vi "CIC_reconfigure_test.vi"() -> ()   [LabVIEW 2013]
uses:
  <vilib>/Analysis/NI_AALBase.lvlib
panel:
  out "Max 2":fxp<+/-,25,19>
  in  "rate":fxp<+,8,8>
  in  "new rate":bool
  out "Array":bool[](array[boolean])
  out "Max Generated":dbl
  out "Simulated":dbl[](graph)
  in  "stop":bool
  out "Filtered":dbl(graph)
  out "Max":fxp<+/-,25,19>
  out "# of Iterations":i32
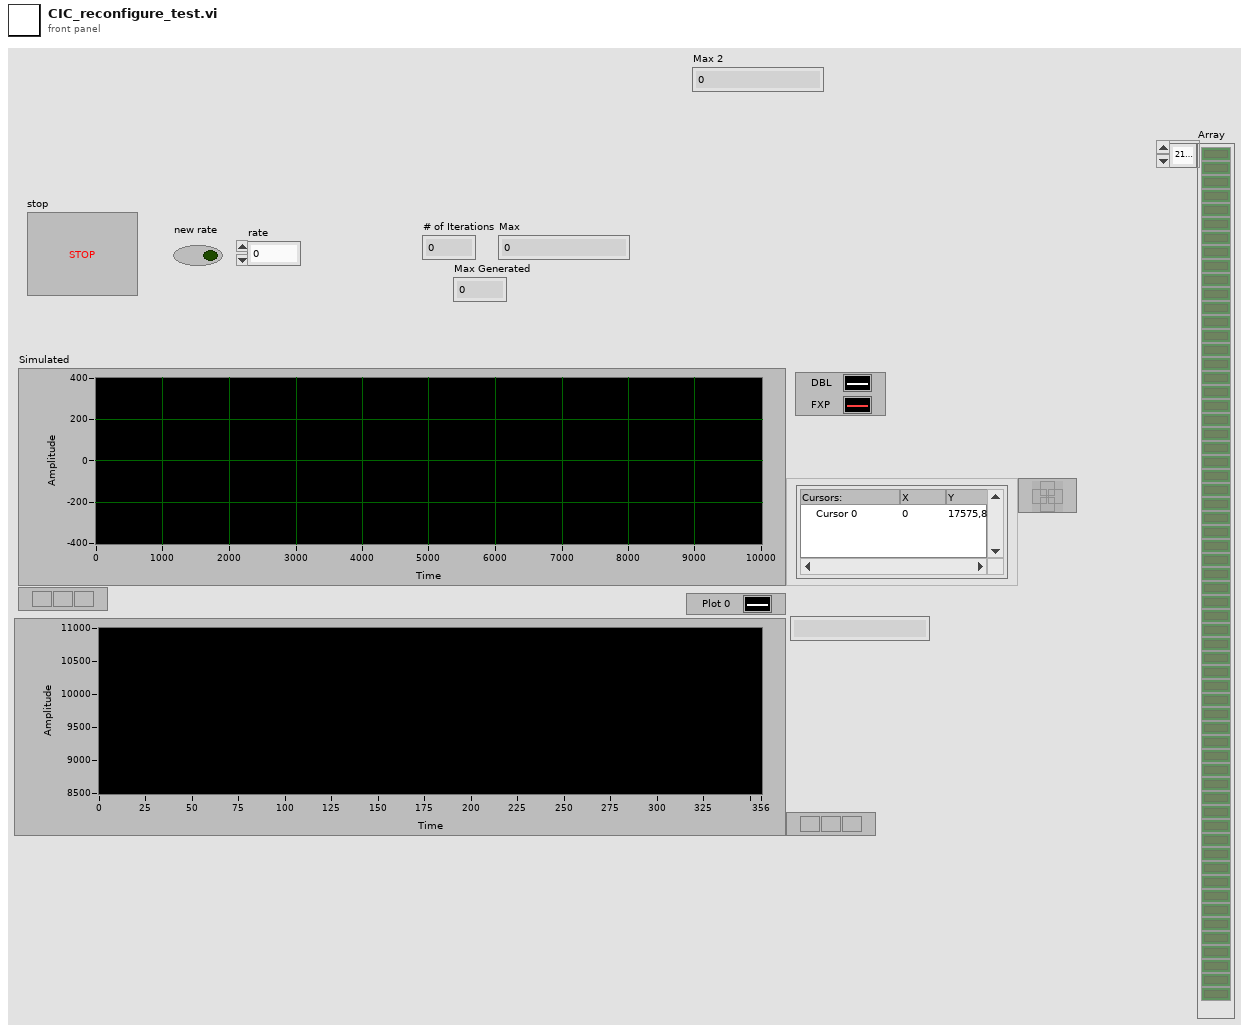
[diagram p1: front panel]
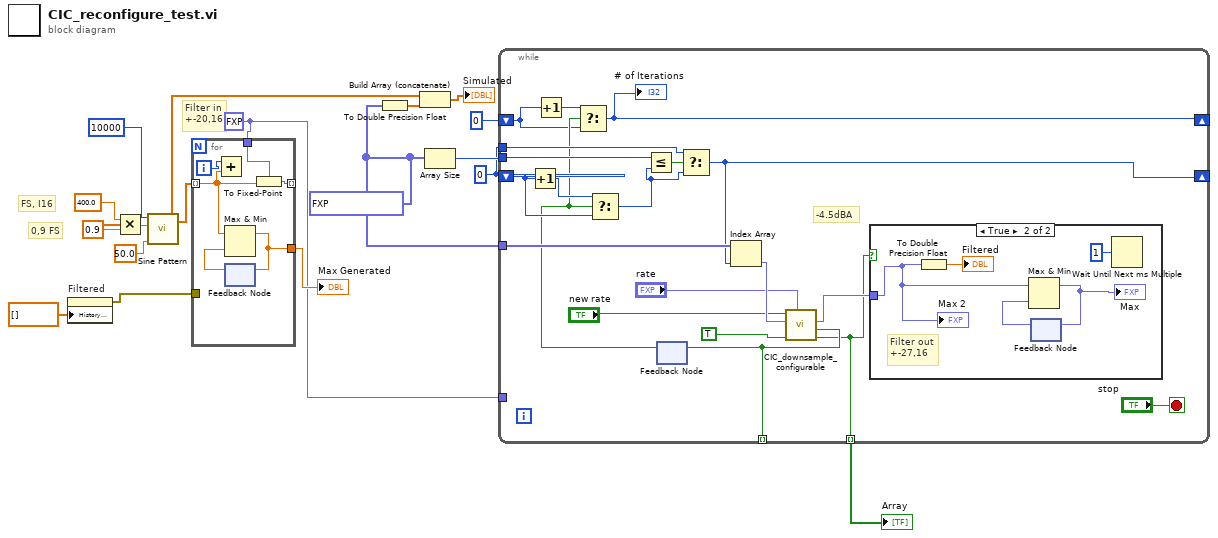
[diagram p0: block diagram]
diagram:
  w1 = fxp<+/-,20,16>[] [100.0]
  w4 = fxp<+/-,20,16> 0.0 ("fixed-point type")
  w12 = 0 ("samples")
  # "Filter in\n+-20,16"
  # "FS, I16"
  # "0,9 FS"
  n1 = property on="Filtered" class="WFChart (strict)"("History Data"=dbl[] []) -> (error out=w6:errorcluster)  [unwired: 2 in, 1 out]
  n2 = Multiply(x=400.0 ("amplitude"), y=0.9) -> (x*y=w14:dbl)
  n3 = call <vilib>:"Sine Pattern.vi"("cycles"=50.0, "amplitude"=w14, "samples"=10000) -> ("Sinusoidal Pattern"=w10:dbl[])  [unwired: 1 in, 1 out]
  n4 = for {
    tunnel: w10 -> [w18] mode=indexing
    tunnel: [w23] -> _ mode=indexing
    tunnel: w4 -> [w22]
    tunnel: [w20] -> w7
    tunnel: w6 -> [_]
    i -> [w19]
    n5 = Add(x=w19, y=w18) -> ()  [unwired: 1 out]
    n6 = feedback #1() -> (w21:dbl)  [unwired: 1 in]
    n7 = Max & Min(x=w18, y=w21) -> (max(x,y)=w20:dbl)  [unwired: 1 out]
    n8 = feedback-in #1(w20) -> ()
    n9 = To Fixed-Point(fixed-point type=w22, number=w18) -> (fixed-point=w23:fxp<+/-,20,16>)
  }
  "Max Generated" <- w7
  n10 = To Double Precision Float(number=w1) -> (double precision float=w11:dbl[])
  n11 = Build Array (concatenate)(w10, w11) -> (→"Simulated":dbl[])
  n12 = Array Size(array=w1) -> (size(s)=w13:i32)
  n13 = while {
    tunnel: w1 -> [w41]
    shift-right: [w40] -> _
    shift-left: w12 -> [w35]
    tunnel: w13 -> [w39]
    tunnel: w12 -> [w42]
    tunnel: w4 -> [_]
    shift-right: [w31] -> _
    shift-left: 0 ("samples") -> [w30]
    tunnel: [w29] -> _ mode=indexing
    tunnel: [w26] -> w2 mode=indexing
    stop <- "stop" stop-if-true
    # "-4.5dBA"
    n14 = Increment(x=w35) -> (x+1=w36:i32)
    n15 = Increment(x=w30) -> (x+1=w32:i32)
    n16 = feedback #2() -> (w33:bool)  [unwired: 1 in]
    n17 = Select(t=w32, s=w33, f=w30) -> (s? t:f=w31:i32)
    "# of Iterations" <- w31
    n18 = Select(t=w36, s=w33, f=w35) -> (s? t:f=w34:i32)
    n19 = Less Or Equal?(x=w39, y=w34) -> (x <= y?=w38:bool)
    n20 = Select(t=w42, s=w38, f=w34) -> (s? t:f=w40:i32)
    n21 = Index Array(array=w41, index=w40) -> (element=w27:fxp<+/-,20,16>)
    n22 = call "CIC_downsample_configurable.vi"("new rate"="rate", "valid in"=TRUE, "din"=w27, "rate change"="new rate") -> ("valid out"=w26:bool, "rdy for data"=w29:bool, "dout"=w28:fxp<+/-,25,19>)  [unwired: 5 in]
    n23 = feedback-in #2(w29) -> ()
    n24 = case shown="True" w26 {
      tunnel: w28 -> [_ w44]
      frame False {
      }
      frame True {
        # "Filter out\n+-27,16"
        n25 = To Double Precision Float(number=w44) -> (double precision float=→"Filtered":dbl)
        n26 = feedback #3() -> (w47:fxp<+/-,25,19>)  [unwired: 1 in]
        n27 = Max & Min(x=w44, y=w47) -> (max(x,y)=w46:fxp<+/-,25,19>)  [unwired: 1 out]
        "Max" <- w46
        n28 = feedback-in #3(w46) -> ()
        n29 = Wait Until Next ms Multiple(millisecond multiple=u32 1) -> ()  [unwired: 1 out]
        "Max 2" <- w44
      }
    }
  }
  "Array" <- w2
